vi "Stop.vi"(8 "error in (no error)":errorcluster, 11 "PID Loop in":refnum<class "PID Loop.lvclass">) -> (0 "error out":errorcluster, 3 "PID Loop out":refnum<class "PID Loop.lvclass">)   [LabVIEW 2024, in "PID Loop.lvlib" / "PID Loop.lvclass"]
uses:
  PID Loop.lvclass
  PID Loop.lvclass/PID Loop.ctl
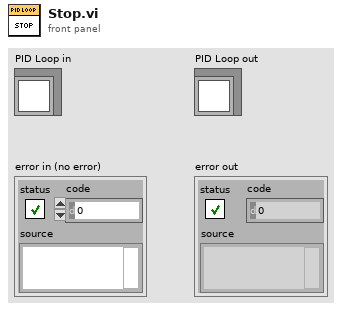
[diagram p1: front panel]
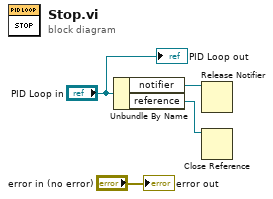
[diagram p0: block diagram]
diagram:
  n1 = Unbundle By Name("PID Loop in") -> ("notifier"=w2:refnum<notifier>, "reference"=w1:refnum<vi>)
  n2 = Release Notifier(notifier=w2) -> ()  [unwired: 2 in, 3 out]
  n3 = Close Reference(reference=w1) -> ()  [unwired: 1 in, 1 out]
  "error out" <- "error in (no error)"
  "PID Loop out" <- "PID Loop in"
